vi "Temp PID v1_0.vi"(1 "Anti-Windup":bool, 2 "Set Point":dbl format="%.3g", 3 "Present Value":dbl format="%.3f", 4 "Tuning Parameters":T1={"Controller Gain, Kc"=1.0, "Reset Time, Ti (s)"=0.01, "Derivative Time, Td (s)"=0.0} {"Derivative Time, Td (s)" format="%.3g"; "Reset Time, Ti (s)" format="%.3g"; "Controller Gain, Kc" format="%.3g"}) -> (0 "Controller Output":dbl format="%.3g")   [LabVIEW 2012]
panel:
  out "dt (min)":dbl format="%.3g"
  in  "dT (s)":dbl=-1.0 step=0.001 format="%.3f"
  # "This PID VI is based on the PID VI  for the  pH controller experiment. It is in ideal form and simplified down from the default NI PID VI."
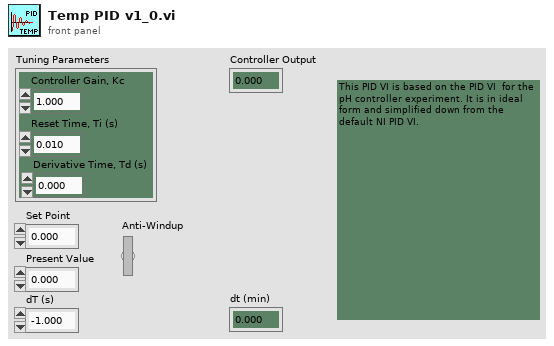
[diagram p1: front panel]
types:
  T1 = cluster{"Controller Gain, Kc":dbl, "Reset Time, Ti (s)":dbl, "Derivative Time, Td (s)":dbl}
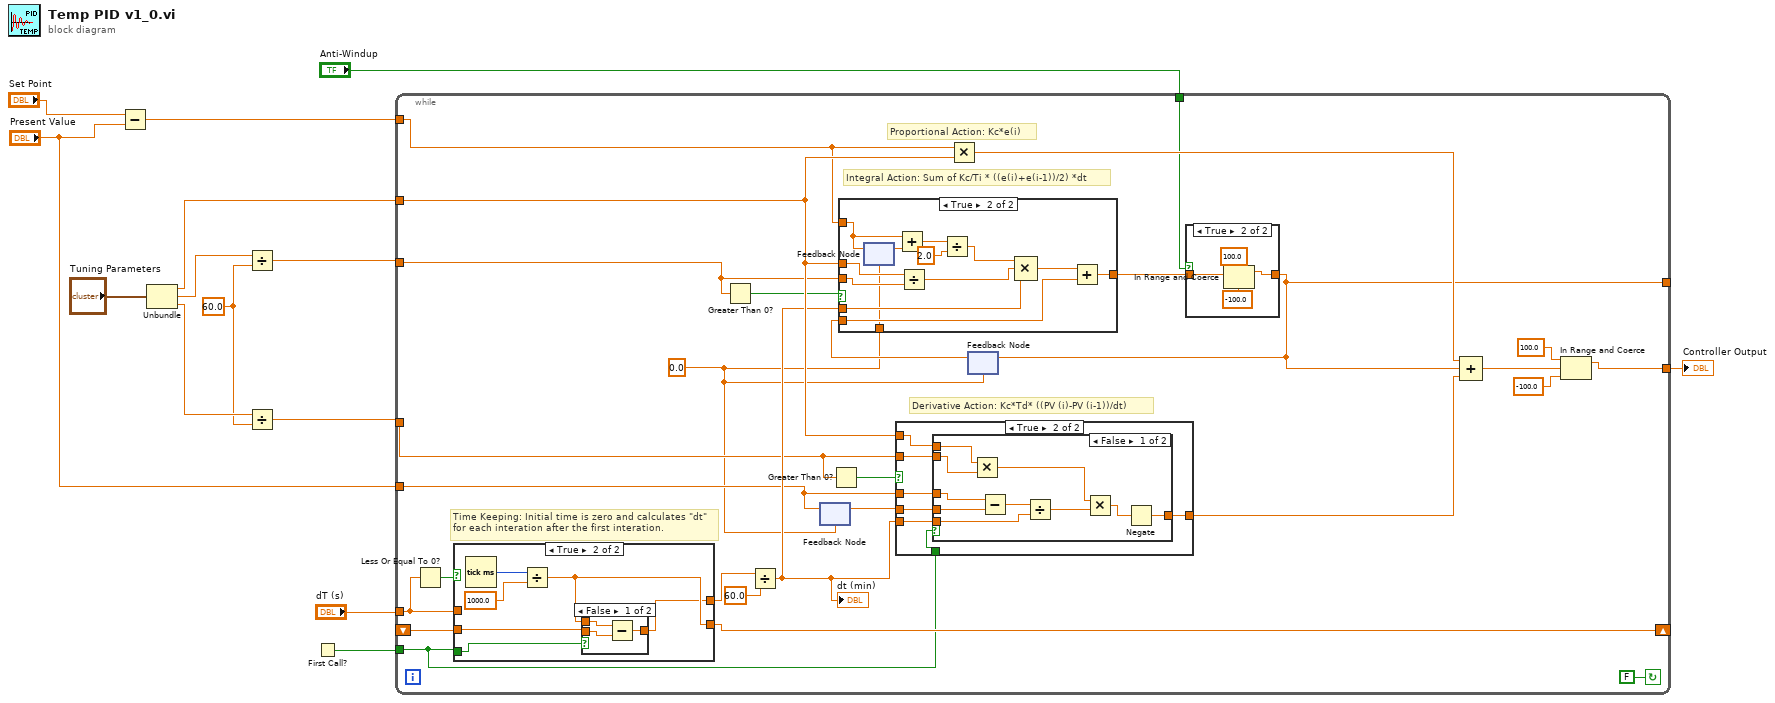
[diagram p0: block diagram]
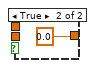
[diagram p4: hidden frame]
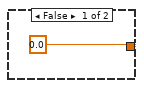
[diagram p5: hidden frame]
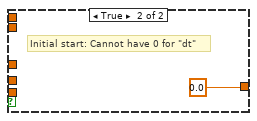
[diagram p6: hidden frame]
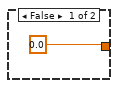
[diagram p7: hidden frame]
diagram:
  w5 = 60.0
  n1 = Subtract(x="Set Point", y="Present Value") -> (x-y=w13:dbl)
  n2 = Unbundle("Tuning Parameters") -> ("Controller Gain, Kc"=w9:dbl, "Reset Time, Ti (s)"=w11:dbl, "Derivative Time, Td (s)"=w10:dbl)
  n3 = Divide(x=w11, y=w5) -> (x/y=w8:dbl)
  n4 = Divide(x=w10, y=w5) -> (x/y=w7:dbl)
  n5 = First Call?() -> (First Call?: T/F=w1:bool)
  n6 = while {
    tunnel: w13 -> [w41]
    tunnel: w9 -> [w42]
    tunnel: w8 -> [w36]
    tunnel: w7 -> [w21]
    tunnel: w1 -> [w24]
    shift-right: [w33] -> _
    shift-left: _ -> [w40]
    tunnel: "dT (s)" -> [w38]
    tunnel: "Present Value" -> [w17]
    tunnel: [w27] -> w3
    tunnel: [w19] -> _
    tunnel: "Anti-Windup" -> [w20]
    stop <- FALSE continue-if-true
    w15 = 0.0
    # "Derivative Action: Kc*Td* ((PV (i)-PV (i-1))/dt)"
    # "Proportional Action: Kc*e(i)"
    # "Integral Action: Sum of Kc/Ti * ((e(i)+e(i-1))/2) *dt"
    # "Time Keeping: Initial time is zero and calculates \"dt\" for each interation after the first interation."
    n7 = Less Or Equal To 0?(x=w38) -> (x <= 0?=w39:bool)
    n8 = case shown="True" w39 {
      tunnel: w24 -> [_ w54]
      tunnel: [w48 w51] -> w33
      tunnel: w40 -> [_ w52]
      tunnel: w38 -> [w48 _]
      tunnel: [w48 w49] -> w32
      frame False {
      }
      frame True {
        n9 = Tick Count (ms)() -> (millisecond timer value=w53:u32)
        n10 = Divide(x=w53, y=1000.0) -> (x/y=w51:dbl)
        n11 = case shown="False" w54 {
          tunnel: w51 -> [w57 _]
          tunnel: w52 -> [w56 _]
          tunnel: [w55 0.0] -> w49
          frame False {
            n12 = Subtract(x=w57, y=w56) -> (x-y=w55:dbl)
          }
          frame True {
          }
        }
      }
    }
    n13 = Greater Than 0?(x=w36) -> (x > 0?=w35:bool)
    n14 = Divide(x=w32, y=60.0) -> (x/y=w37:dbl)
    "dt (min)" <- w37
    n15 = feedback #1(w15) -> (w16:dbl)
    n16 = feedback-in #1(w17) -> ()
    n17 = Greater Than 0?(x=w21) -> (x > 0?=w26:bool)
    n18 = case shown="True" w26 {
      tunnel: w42 -> [_ w64]
      tunnel: w21 -> [_ w63]
      tunnel: w37 -> [_ w65]
      tunnel: w17 -> [_ w66]
      tunnel: [0.0 w62] -> w34
      tunnel: w24 -> [_ w61]
      tunnel: w16 -> [_ w60]
      frame False {
      }
      frame True {
        n19 = case shown="False" w61 {
          tunnel: w66 -> [w76 _]
          tunnel: w65 -> [w74 _]
          tunnel: w64 -> [w73 _]
          tunnel: w63 -> [w72 _]
          tunnel: [w68 0.0] -> w62
          tunnel: w60 -> [w67 _]
          frame False {
            n20 = Multiply(x=w73, y=w72) -> (x*y=w71:dbl)
            n21 = Subtract(x=w76, y=w67) -> (x-y=w75:dbl)
            n22 = Divide(x=w75, y=w74) -> (x/y=w70:dbl)
            n23 = Multiply(x=w71, y=w70) -> (x*y=w69:dbl)
            n24 = Negate(x=w69) -> (-x=w68:dbl)
          }
          frame True {
            # "Initial start: Cannot have 0 for \"dt\""
          }
        }
      }
    }
    n25 = Multiply(x=w41, y=w42) -> (x*y=w23:dbl)
    n26 = feedback #2(w15) -> (w18:dbl)
    n27 = case shown="True" w35 {
      tunnel: w42 -> [_ w89]
      tunnel: w36 -> [_ w88]
      tunnel: w41 -> [_ w82]
      tunnel: w37 -> [_ w85]
      tunnel: [0.0 w83] -> w22
      tunnel: w18 -> [_ w80]
      tunnel: w15 -> [_ w79]
      frame False {
      }
      frame True {
        n28 = feedback #3(w79) -> (w81:dbl)
        n29 = feedback-in #3(w82) -> ()
        n30 = Add(x=w82, y=w81) -> (x+y=w91:dbl)
        n31 = Divide(x=w89, y=w88) -> (x/y=w86:dbl)
        n32 = Divide(x=w91, y=2.0) -> (x/y=w87:dbl)
        n33 = Compound Arithmetic op=MULTIPLY(w87, w86, w85) -> (w84:dbl)
        n34 = Add(x=w84, y=w80) -> (x+y=w83:dbl)
      }
    }
    n35 = case shown="True" w20 {
      tunnel: w22 -> [w43 w47]
      tunnel: [w43 w46] -> w19
      frame False {
      }
      frame True {
        n36 = In Range and Coerce(upper limit=100.0 ("lower limit"), x=w47, lower limit=-100.0) -> (coerced(x)=w46:dbl)  [unwired: 1 out]
      }
    }
    n37 = feedback-in #2(w19) -> ()
    n38 = Compound Arithmetic op=ADD(w23, w19, w34) -> (w28:dbl)
    n39 = In Range and Coerce(upper limit=100.0 ("x"), x=w28, lower limit=-100.0 ("x")) -> (coerced(x)=w27:dbl)  [unwired: 1 out]
  }
  "Controller Output" <- w3
